vi "test_InitializeItemContents.vi"() -> (2 "Actuals":T1[](array[typedef]), 3 "Pass?":bool)   [LabVIEW 2020, in "Tests.LabVIEWItem.lvlib"]
uses:
  Validation/Validate_BaseConstruction.ctl
  CLabVIEWItem/CLabVIEWItem.lvclass
  Tests.LabVIEWItem.lvlib
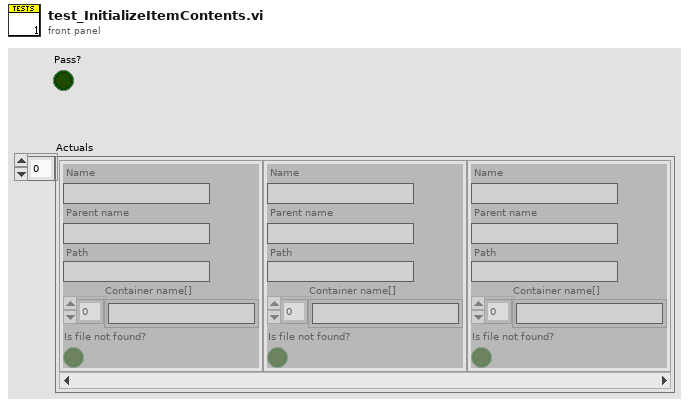
[diagram p1: front panel]
types:
  T1 = typedef "Tests.LabVIEWItem.lvlib/Validate_BaseConstruction.ctl" = cluster{"Name":string, "Parent name":string, "Path":string, "Container name[]":string[], "Is file not found?":bool}
  T2 = typedef "Tests.LabVIEWItem.lvlib/Params_ConstructLabVIEWItem.ctl" = cluster{"Input":T3, "Validation":T1}
  T3 = typedef "Tests.LabVIEWItem.lvlib/Input_BaseConstruction.ctl" = cluster{"Qualified name":string, "Path":string, "Error code":i32}
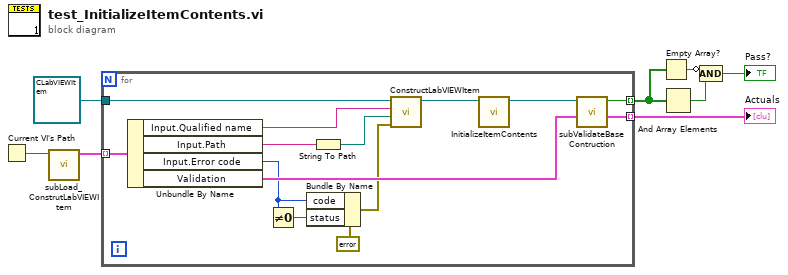
[diagram p0: block diagram]
diagram:
  n1 = Current VI's Path() -> (path=w7:path)
  n2 = call "subLoad_ConstrutLabVIEWItem.vi"("Caller path"=w7) -> ("Params"=w6:T2[])  [unwired: 10 in]
  n3 = for {
    tunnel: refnum<class "CLabVIEWItem.lvclass"> refnum ("CLabVIEWItem in") -> [w22]
    tunnel: [w21] -> w1 mode=indexing
    tunnel: w6 -> [w19] mode=indexing
    tunnel: [w20] -> w5 mode=indexing
    n4 = Unbundle By Name(w19) -> ("Input.Qualified name"=w17:string, "Input.Path"=w16:string, "Input.Error code"=w12:i32, "Validation"=w18:T1)
    n5 = Not Equal To 0?(x=w12) -> (x != 0?=w11:bool)
    n6 = Bundle By Name(cluster=errorcluster {"status"=FALSE, "code"=0, "source"=""} ("error in (no error)"), "code"=w12, "status"=w11) -> (w13:errorcluster)
    n7 = String To Path(string=w16) -> (path=w15:path)
    n8 = call-dynamic "ConstructLabVIEWItem.vi"("error in (no error)"=w13, "Path"=w15, "Qualified name"=w17, "CLabVIEWItem in"=w22) -> ("CLabVIEWItem out"=w10:refnum<class "CLabVIEWItem.lvclass">)  [unwired: 6 in, 1 out]
    n9 = call-dynamic "InitializeItemContents.vi"("CLabVIEWItem in"=w10) -> ("CLabVIEWItem out"=w9:refnum<class "CLabVIEWItem.lvclass">)  [unwired: 9 in, 1 out]
    n10 = call "subValidateBaseContruction.vi"("Parameters"=w18, "CLabVIEWItem in"=w9) -> ("Actual"=w21:T1, "Pass?"=w20:bool)  [unwired: 8 in]
  }
  "Actuals" <- w1
  n11 = Empty Array?(array=w5) -> (empty?=w4:bool)
  n12 = And Array Elements(Boolean array=w5) -> (logical AND=w3:bool)
  n13 = Compound Arithmetic op=AND(invert w4, w3) -> (→"Pass?":bool)
